vi "PowerTransformer.vi"(8 "error in (no error)":errorcluster caption="entrée d'erreur (pas d'erreur)", 11 "PowerTransformer":T1={"method"="yeo-johnson", "standardize"=TRUE, "copy"=TRUE}) -> (0 "error out":errorcluster, 3 "PowerTransformer.lvclass":refnum<class "PowerTransformer.lvclass">)   [LabVIEW 2020]
doc: "Apply a power transform featurewise to make data more Gaussian-like.\n\nPower transforms are a family of parametric, monotonic transformations that are applied to make data more Gaussian-like. This is useful for modeling issues related to heteroscedasticity (non-constant variance), or other situations where normality is desired.\n\nCurrently, PowerTransformer supports the Box-Cox transform and the Yeo-Johnson transform. The optimal parameter for stabilizing variance and minimizing skewness is estimated through maximum likelihood.\n\nBox-Cox requires input data to be strictly positive, while Yeo-Johnson supports both positive or negative data.\n\nBy default, zero-mean, unit-variance normalization is applied to the transformed data.\n\n\nParameters : \n\n- method : str, (default=’yeo-johnson’)\nThe power transform method. Available methods are:\n\n‘yeo-johnson’, works with positive and negative values\n\n‘box-cox’, only works with strictly positive values\n\n- standardize : boolean, default=True\nSet to True to apply zero-mean, unit-variance normalization to the transformed output.\n\n- copy : boolean, optional, default=True\nSet to False to perform inplace computation during transformation.\n\n\nMethods : \n\n\n- Fit : Estimate the optimal parameter lambda for each feature. The optimal lambda parameter for minimizing skewness is estimated on each feature independently using maximum likelihood.\n\nParameters : X : array-like, shape (n_samples, n_features)\n The data used to estimate the optimal transformation parameters.\n y : Ignored\n\n\n- Fit Transform : Fit to data, then transform it. Fits transformer to X and y with optional parameters fit_params and returns a transformed version of X.\n\nParameters : X : {array-like, sparse matrix, dataframe} of shape (n_samples, n_features)\n y : ndarray of shape (n_samples,), default=None\n Target values.\n\nReturns : X_new : ndarray array of shape (n_samples, n_features_new)\n Transformed array.\n\n\n- Transform : Apply the power transform to each feature using the fitted lambdas.\n\nParameters : X : array-like, shape (n_samples, n_features)\n The data to be transformed using a power transformation.\n\nReturns : X_trans : array-like, shape (n_samples, n_features)\n The transformed data."
uses:
  PowerTransformer.lvclass
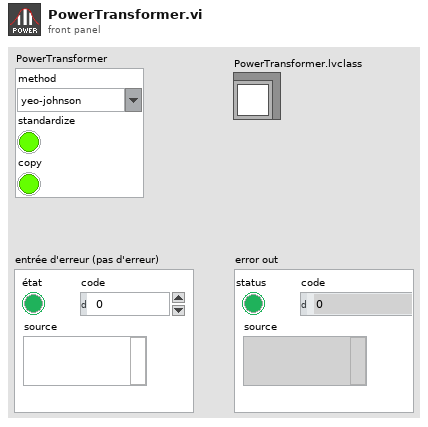
[diagram p1: front panel]
types:
  T1 = cluster{"method":string, "standardize":bool, "copy":bool}
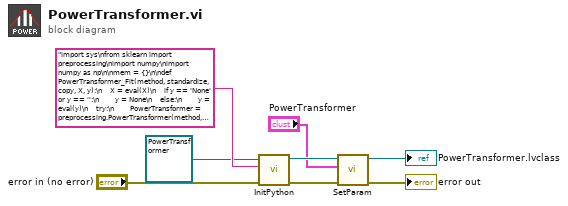
[diagram p0: block diagram]
diagram:
  n1 = call-dynamic "InitPython.vi"("error in (no error)"="error in (no error)", "Python Instruction"="import sys\nfrom sklearn import preprocessing\nimport numpy\nimport numpy as np\n\nmem = {}\n\ndef PowerTransformer_Fit(method, standardize, copy, X, y):\n    X = eval(X)\n    if y == 'None' or y == '':\n        y = None\n    else:\n        y = eval(y)\n    try:\n        PowerTransformer = preprocessing.PowerTransformer(method, standardize, copy).fit(X, y)\n        mem['FitPowerTransformer'] = PowerTransformer\n        return str('OK')\n    except:\n        erreur = sys.exc_info()\n        typerr = u\"%s\" % (erreur[0])\n        typerr = typerr[typerr.find(\"'\")+1:typerr.rfind(\"'\")]\n        msgerr = u\"%s\" % (erreur[1])\n        message = str('/!\\\\ {0} : {1}'. format(typerr,msgerr))\n        return message \n    \ndef PowerTransformer_FitTransform(method, standardize, copy, X, y):\n    X = eval(X)\n    if y == 'None' or y == '':\n        y = None\n    else:\n        y = eval(y)\n    try:\n        PowerTransformer = preprocessing.PowerTransformer(method, standardize, copy).fit_transform(X, y)\n        dtype = type(PowerTransformer)\n        if dtype == numpy.ndarray:\n            PowerTransformer = PowerTransformer.tolist()\n            return str(PowerTransformer) \n        else:\n            Mat = PowerTransformer.tocoo()\n            return str(list(zip(Mat.row, Mat.col, Mat.data)))\n    except:\n        erreur = sys.exc_info()\n        typerr = u\"%s\" % (erreur[0])\n        typerr = typerr[typerr.find(\"'\")+1:typerr.rfind(\"'\")]\n        msgerr = u\"%s\" % (erreur[1])\n        message = str('/!\\\\ {0} : {1}'. format(typerr,msgerr))\n        return message \n\ndef PowerTransformer_Transform(method, standardize, copy, X, y):\n    X = eval(X)\n    if y == 'None' or y == '':\n        y = None\n    else:\n        y = eval(y)\n    try:\n        PowerTransformer = mem['FitPowerTransformer'].transform(X)\n        dtype = type(PowerTransformer)\n        if dtype == numpy.ndarray:\n            PowerTransformer = PowerTransformer.tolist()\n            return str(PowerTransformer) \n        else:\n            Mat = PowerTransformer.tocoo()\n            return str(list(zip(Mat.row, Mat.col, Mat.data)))\n    except:\n        erreur = sys.exc_info()\n        typerr = u\"%s\" % (erreur[0])\n        typerr = typerr[typerr.find(\"'\")+1:typerr.rfind(\"'\")]\n        msgerr = u\"%s\" % (erreur[1])\n        message = str('/!\\\\ {0} : {1}'. format(typerr,msgerr))\n        return message", "Scikit-learn en entrée"=refnum<class "PowerTransformer.lvclass"> refnum ("PowerTransformer.lvclass")) -> ("error out"=w3:errorcluster, "Scikit-learn en sortie"=w5:refnum<class "PowerTransformer.lvclass">)  [unwired: 7 in]
  n2 = call-dynamic "SetParam.vi"("error in (no error)"=w3, "PowerTransformer"="PowerTransformer", "PowerTransformer.lvclass"=w5) -> ("error out"=→"error out":errorcluster, "PowerTransformer.lvclass"=→"PowerTransformer.lvclass":refnum<class "PowerTransformer.lvclass">)  [unwired: 7 in]
